vi "testOutsideRoot.vi"(8 "error in (no error)":errorcluster, 11 "TestCase in":refnum<class "LocationOutsideClassRoot.lvclass">) -> (0 "error out":errorcluster, 3 "TestCase out":refnum<class "LocationOutsideClassRoot.lvclass">)   [LabVIEW 2013, in "LocationOutsideClassRoot.lvclass"]
uses:
  LocationOutsideClassRoot.lvclass
  Classes/TestCase/TestCase.lvclass
panel:
  # "Copyright © 2007 James Kring, Inc. All rights reserved.\n\nAuthor: Jim Kring [jim.kring@jameskring.com]\n\nThis library is provided \"AS IS\" ,WITHOUT WARRANTIES OR \nCONDITIONS OF ANY KIND, either express or implied.\n\nJames Kring, Inc. -- http://www.jameskring.com"
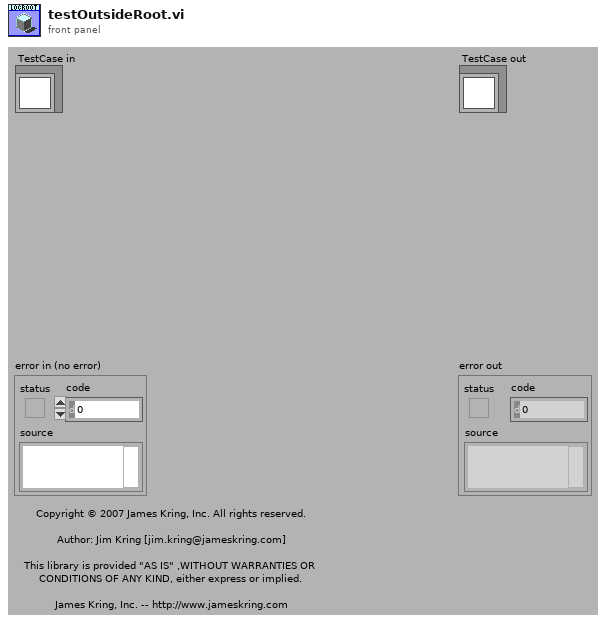
[diagram p1: front panel]
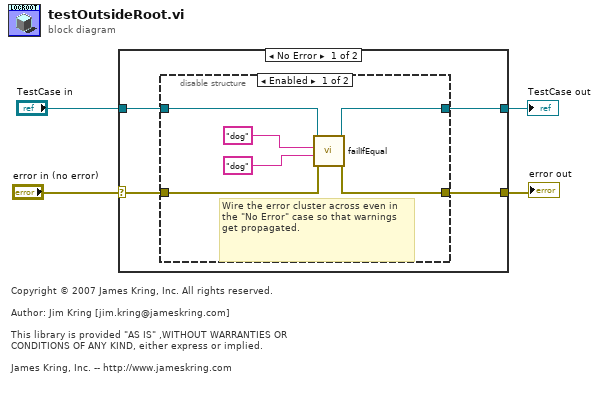
[diagram p0: block diagram]
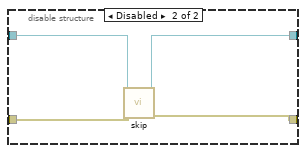
[diagram p2: hidden frame]
diagram:
  # "Copyright © 2007 James Kring, Inc. All rights reserved.\n\nAuthor: Jim Kring [jim.kring@jameskring.com]\n\nThis library is provided \"AS IS\" ,WITHOUT WARRANTIES OR \nCONDITIONS OF ANY KIND, either express or implied.\n\nJames Kring, Inc. -- http://www.jameskring.com"
  n1 = case shown="No Error" "error in (no error)" {
    selector: "error in (no error)" -> [w6 w20]
    tunnel: [w5 w20] -> w3
    tunnel: [w7 w19] -> w1
    tunnel: "TestCase in" -> [w8 w19]
    frame No Error {
      n2 = disable-structure shown="Enabled" {
        disable-tunnel: w8 -> [w12 w16]
        disable-tunnel: [w11 w15] -> w7
        disable-tunnel: w6 -> [w10 w18]
        disable-tunnel: [w9 w17] -> w5
        frame Enabled {
          # "Wire the error cluster across even in the \"No Error\" case so that warnings get propagated."
          n3 = call-dynamic "failIfEqual.vi"("error in (no error)"=w10, "y"="dog", "x"="dog", "TestCase in"=w12) -> ("error out"=w9:errorcluster, "TestCase out"=w11:refnum<class "LocationOutsideClassRoot.lvclass">)  [unwired: 6 in]
        }
        frame Disabled {
          n4 = call "skip.vi"("error in (no error)"=w18, "TestCase in"=w16) -> ("error out"=w17:errorcluster, "TestCase out"=w15:refnum<class "LocationOutsideClassRoot.lvclass">)  [unwired: 8 in]
        }
      }
    }
    frame Error {
    }
  }
  "error out" <- w3
  "TestCase out" <- w1
